vi "PSVCH_DBL String Check.vi"(10 "Num Str":string) -> (1 "Number":dbl, 2 "Num?":bool)   [LabVIEW 2016]
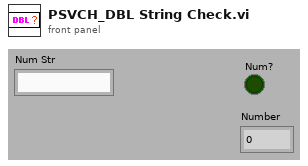
[diagram p1: front panel]
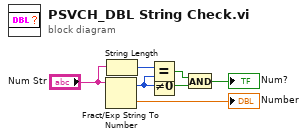
[diagram p0: block diagram]
diagram:
  n1 = Fract/Exp String To Number(string="Num Str") -> (offset past number=w5:i32, number=→"Number":dbl)  [unwired: 3 in]
  n2 = String Length(string="Num Str") -> (length=w6:i32)
  n3 = Equal?(x=w6, y=w5) -> (x = y?=w3:bool)
  n4 = Not Equal To 0?(x=w5) -> (x != 0?=w4:bool)
  n5 = And(x=w3, y=w4) -> (x .and. y?=→"Num?":bool)
